vi "Fetch Single Record Single Channel(4xI16).vi"(7 "Timeout (s)":i32=5, 8 "error in":errorcluster, 11 "FPGA VI Reference In":refnum<k20>) -> (0 "error out":errorcluster, 2 "Acquired Data":i16[](array[numeric]), 3 "FPGA VI Reference Out":refnum<k20>)   [LabVIEW 2012]
uses:
  <vilib>/Utility/error.llb/Error Cluster From Error Code.vi
  <vilib>/rvi/errors/niLvFpgaAdjustHostInterfaceError.vi
  <vilib>/rvi/interface/nirviReadWriteControl/nirviReadWriteControl.xnode
  NiFpgaLv.dll
  <vilib>/rvi/interface/Simulation/niFpgaSimulationCallBeginRW.vi
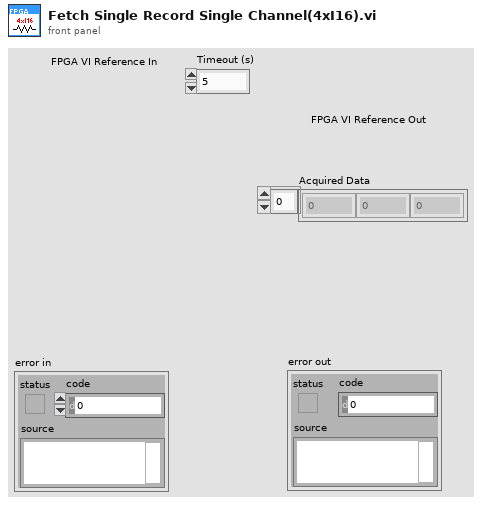
[diagram p1: front panel]
types:
  T1 = cluster{"Load Record Parameters?":bool, "Pre Trigger Samples":u16, "Samples per Record":u16, "Trigger Hold Off":u16, "Record Count":u16}
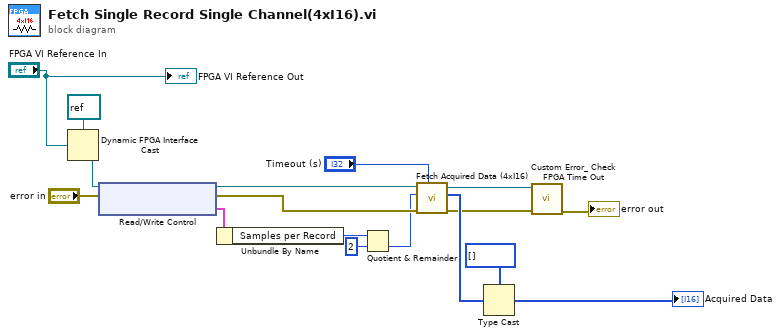
[diagram p0: block diagram]
diagram:
  n1 = Dynamic FPGA Interface Cast(Session In=refnum<k20> refnum ("Type"), Type="FPGA VI Reference In") -> (Session Out=w14:refnum<k20>)
  n2 = xnode "Read/Write Control"("FPGA VI Reference In"=w14, "error in"="error in") -> ("FPGA VI Reference Out"=w11:refnum<k20>, "error out"=w10:errorcluster, "Record Parameters"=w13:T1)
  n3 = Unbundle By Name(w13) -> ("Samples per Record"=w12:u16)
  n4 = Quotient & Remainder(x=w12, y=u16 2) -> (floor(x/y)=w2:u16)  [unwired: 1 out]
  n5 = call <userlib>:"Fetch Acquired Data (4xI16).vi"("Timeout (s)"="Timeout (s)", "error out"=w10, "Samples"=w2, "FPGA Ref In"=w11) -> ("error out"=w5:errorcluster, "Data"=w8:i16[], "FPGA RefOut"=w6:refnum<k20>)  [unwired: 4 in, 1 out]
  n6 = Type Cast(type=i16[] [], x=w8) -> (*(type *) &x=→"Acquired Data":i16[])
  n7 = call <userlib>:"Custom Error_ Check FPGA Time Out.vi"("error in"=w5, "FPGA VI Reference In"=w6) -> ("error out"=→"error out":errorcluster)  [unwired: 8 in, 1 out]
  "FPGA VI Reference Out" <- "FPGA VI Reference In"
